vi "proj_czyszczenie_graj.vi"(6 "Table control 4":refnum<vi>, 7 "Przycisk":bool, 10 "Table control 2":refnum<vi>, 11 "Table control 1":refnum<vi>) -> ()   [LabVIEW 2020]
uses:
  <vilib>/Utility/miscctls.llb/LVRowAndColumnTypeDef.ctl
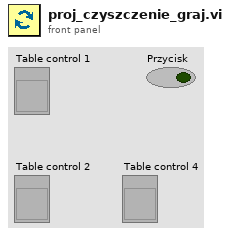
[diagram p1: front panel]
types:
  T1 = typedef "LVRowAndColumnTypeDef.ctl" = cluster{"Row":i32, "Column":i32}
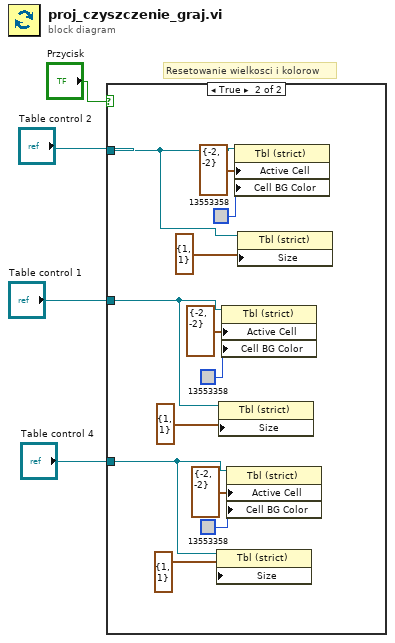
[diagram p0: block diagram]
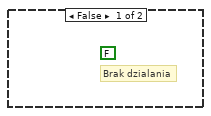
[diagram p2: hidden frame]
diagram:
  # "Resetowanie wielkosci i kolorow"
  n1 = case shown="True" "Przycisk" {
    tunnel: "Table control 1" -> [_ w7]
    tunnel: "Table control 2" -> [_ w9]
    tunnel: "Table control 4" -> [_ w5]
    frame False {
      (unwired) FALSE
      # "Brak dzialania"
    }
    frame True {
      n2 = property on="Property Node" class="Tbl (strict)"(reference=w5, "Size"=cluster{"Row":i32, "Column":i32} {"Row"=1, "Column"=1} ("Edit Position")) -> ()  [unwired: 1 in, 2 out]
      n3 = property on="Property Node" class="Tbl (strict)"(reference=w7, "Size"=cluster{"Row":i32, "Column":i32} {"Row"=1, "Column"=1} ("Edit Position")) -> ()  [unwired: 1 in, 2 out]
      n4 = property on="Property Node" class="Tbl (strict)"(reference=w7, "Active Cell"=T1 {"Row"=-2, "Column"=-2} ("Active Cell:Active Cell"), "Cell BG Color"=u32 13553358 ("Active Cell:Cell Background Color")) -> ()  [unwired: 1 in, 2 out]
      n5 = property on="Property Node" class="Tbl (strict)"(reference=w5, "Active Cell"=T1 {"Row"=-2, "Column"=-2} ("Active Cell:Active Cell"), "Cell BG Color"=u32 13553358 ("Active Cell:Cell Background Color")) -> ()  [unwired: 1 in, 2 out]
      n6 = property on="Property Node" class="Tbl (strict)"(reference=w9, "Active Cell"=T1 {"Row"=-2, "Column"=-2} ("Active Cell:Active Cell"), "Cell BG Color"=u32 13553358 ("Active Cell:Cell Background Color")) -> ()  [unwired: 1 in, 2 out]
      n7 = property on="Property Node" class="Tbl (strict)"(reference=w9, "Size"=cluster{"Row":i32, "Column":i32} {"Row"=1, "Column"=1} ("Edit Position")) -> ()  [unwired: 1 in, 2 out]
    }
  }
